vi "Magnetic Sweep 1.7.vi"() -> ()   [LabVIEW 2011]
uses:
  <vilib>/Math Plots/3D Math Plots/3D Scatter/3D Scatter XCtrl/3D Scatter.xctl
  <vilib>/Math Plots/3D Math Plots/3D Scatter/3D Scatter Datatype/Public/Plot Helper (Vector).vi
  <vilib>/Math Plots/3D Math Plots/3D Scatter/3D Scatter Datatype/3D Scatter Datatype.lvclass
panel:
  out "3D Scatter\n(ramp up)":refnum<class "3D Plot Datatype.lvclass">[](xcontrol)
  out "3D Scatter\n(ramp down)":refnum<class "3D Plot Datatype.lvclass">[](xcontrol)
  out "Heater":bool
  out "Persistent switch ready":bool
  out "error out 6":errorcluster
  in  "Temperature\nlower limite":dbl
  out "Ramping rate command":string
  out "Target field command":string
  out "error out 5":errorcluster
  in  "error out 4":errorcluster
  out "String":string="Persistent switch is not on"
  in  "Set parameter":bool
  out "status":string
  out "PID command":string
  out "setpoint command":string
  out "setpoint":dbl
  in  "stop":bool
  out "error out 3":errorcluster
  out "error out 2":errorcluster
  in  "Contour plot (ramp down)":path
  in  "Raw data (ramp down)":path
  out "Elapsed Time (s)":dbl
  out "Iteration":i32
  in  "error out":errorcluster
  out "Initial Temperature":string
  out "Zero field reached":bool
  out "Target field reached":bool
  in  "Temperature\nupper limite":dbl
  in  "Temperature\nramping step":dbl
  in  "Heater range":i16(ring) items=["High", "Medium", "Low"]
  in  "D gain":dbl
  in  "I gain":dbl
  in  "P gain":dbl
  in  "Contour plot (ramp up)":path
  out "Time elapsed":string
  in  "Timer":bool caption="Reset"
  in  "date format":enum16{"short", "long", "abbreviated"}(ring)
  in  "Save":bool
  in  "Raw data (ramp  up)":path
  out "Temperature vs Time":cluster{dbl[], dbl[]}(graph)
  out "current time":timestamp
  out "Magnetic\nField":cluster{dbl[], dbl[]}(graph)
  out "Current Resistance":string
  out "Current Temperature":string
  out "Current Field":string
  out "Status":string
  in  "Field Sweep":bool
  in  "Magnetic field\nRamp rate":dbl
  in  "Traget Field":dbl
  out "Init Response":string
  in  "error in (no error)":errorcluster
  in  "IP Address":string
  in  "Ramp":bool
  in  "Update":bool
  in  "Ramp to Zero":bool
  in  "P Switch":bool
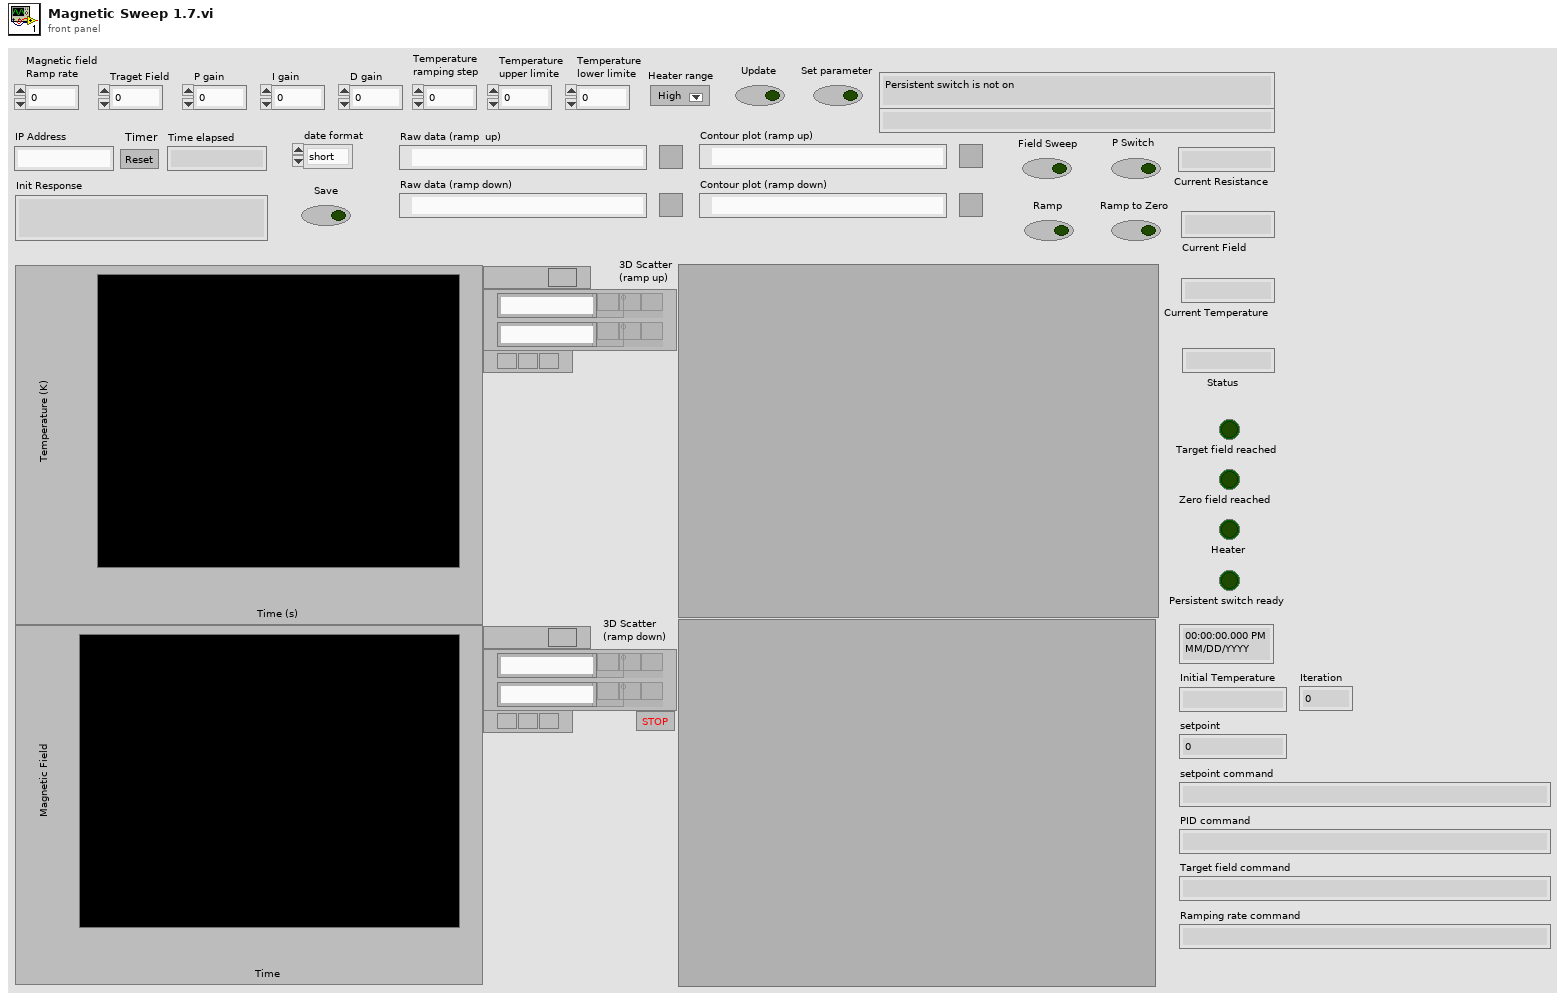
[diagram p1: front panel]
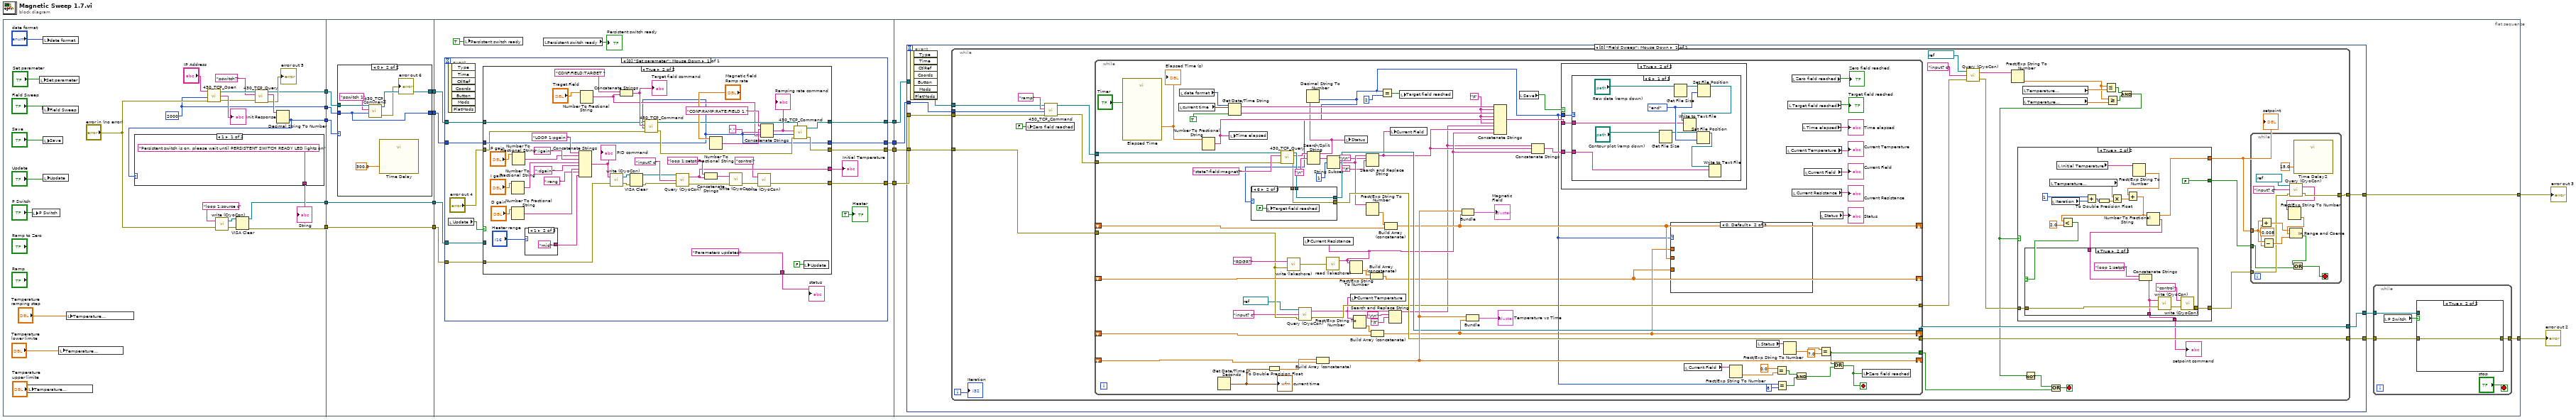
[diagram p0: block diagram]
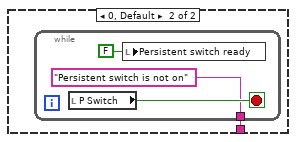
[diagram p2: hidden frame]
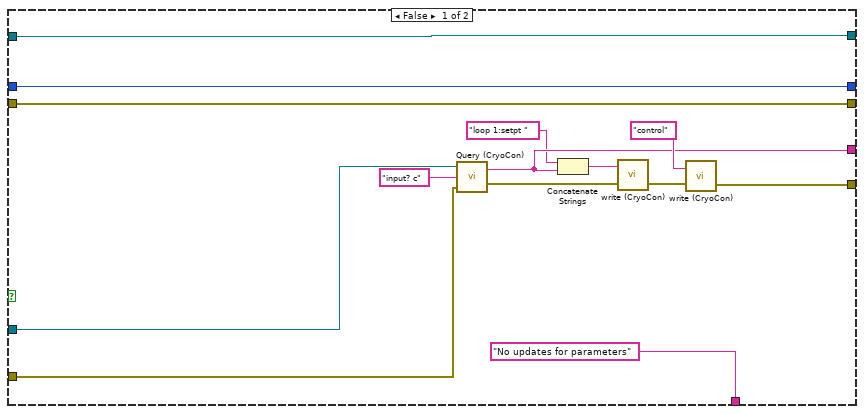
[diagram p4: hidden frame]
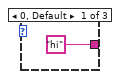
[diagram p5: hidden frame]
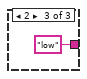
[diagram p6: hidden frame]
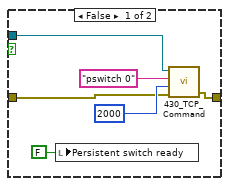
[diagram p7: hidden frame]
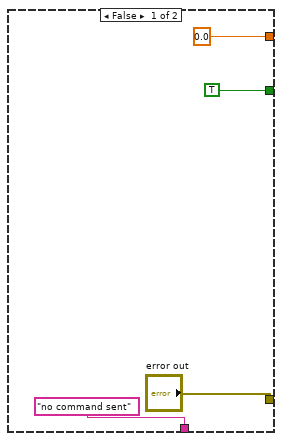
[diagram p8: hidden frame]
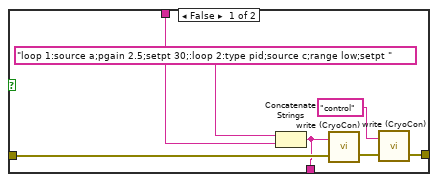
[diagram p9: hidden frame]
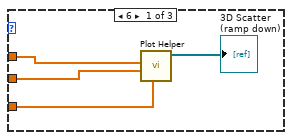
[diagram p10: hidden frame]
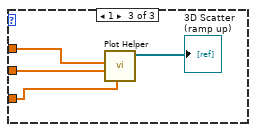
[diagram p11: hidden frame]
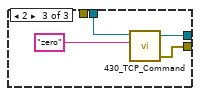
[diagram p13: hidden frame]
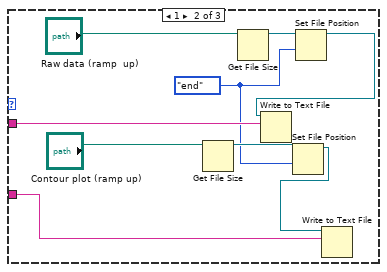
[diagram p15: hidden frame]
diagram:
  n1 = flat-sequence {
    tunnel: [w17] -> w9
    tunnel: [w20] -> w7
    tunnel: [w23] -> w5
    tunnel: [w21] -> w3
    tunnel: [w16] -> w1
    tunnel: w9 -> [w51]
    tunnel: [w49] -> w8
    tunnel: w7 -> [w50]
    tunnel: [w47] -> w6
    tunnel: w5 -> [w53]
    tunnel: [w53] -> w4
    tunnel: w3 -> [w52]
    tunnel: [w52] -> w2
    tunnel: w1 -> [w48]
    tunnel: w8 -> [w62]
    tunnel: w6 -> [w71]
    tunnel: w4 -> [w70]
    tunnel: [w69] -> w15
    tunnel: [w68] -> w12
    tunnel: [w67] -> w11
    tunnel: [w66] -> w10
    tunnel: w2 -> [w65]
    tunnel: w15 -> [w153]
    tunnel: [w152] -> w14
    tunnel: [w150] -> w13
    tunnel: w12 -> [w148]
    tunnel: w11 -> [w147]
    tunnel: w10 -> [w146]
    frame #0 {
      w20 = 2000 ("Timeout")
      n2 = local write "Temperature\nupper limite"("Temperature\nupper limite") -> ()
      n3 = local write "P Switch"("P Switch") -> ()
      n4 = local write "Set parameter"("Set parameter") -> ()
      n5 = local write "date format"("date format") -> ()
      n6 = local write "Field Sweep"("Field Sweep") -> ()
      n7 = local write "Save"("Save") -> ()
      n8 = local write "Update"("Update") -> ()
      n9 = local write "Temperature\nlower limite"("Temperature\nlower limite") -> ()
      n10 = local write "Temperature\nramping step"("Temperature\nramping step") -> ()
      n11 = call "430_TCP_Open.vi"("IP Address"="IP Address", "timeout ms (2000)"=w20, "error in (no error)"="error in (no error)") -> ("connection ID"=w30:refnum<k5>, "Init Response"=→"Init Response":string, "error out"=w29:errorcluster)  [unwired: 3 in]
      n12 = call "write (CryoCon).vi"("error in (no error)"="error in (no error)", "write buffer"="loop 1:source c") -> ("error out"=w25:errorcluster, "VISA resource name out"=w24:refnum<visa-resource-name>)
      n13 = VISA Clear(VISA resource name=w24, error in (no error)=w25) -> (VISA resource name out=w21:refnum<visa-resource-name>, error out=w23:errorcluster)
      n14 = call "430_TCP_Query.vi"("error in (no error)"=w29, "Command"="pswitch?", "connection ID"=w30) -> ("error out"=→"error out 5":errorcluster, "Response"=w27:string, "connection ID out"=w17:refnum<k5>)  [unwired: 4 in, 2 out]
      n15 = Decimal String To Number(string=w27) -> (number=w16:i32)  [unwired: 2 in, 1 out]
      n16 = case shown="1" w16 {
        tunnel: ["Persistent switch is on, please wait until PERSISTENT SWITCH READY LED lights on" w43] -> w22
        frame 1 {
        }
        frame 0, Default {
          n17 = while {
            tunnel: ["Persistent switch is not on"] -> w43
            stop <- w46 stop-if-true
            n18 = local read "P Switch"() -> (w46:bool)
            n19 = local write "Persistent switch ready"(FALSE ("Persistent switch ready")) -> ()
          }
        }
      }
      "String" <- w22
    }
    frame #1 {
      n20 = case shown="0" w48 {
        tunnel: w51 -> [w55 w61]
        tunnel: w50 -> [w54 w56]
        tunnel: [w55 w60] -> w49
        tunnel: [w54 w56] -> w47
        frame 1, Default {
        }
        frame 0 {
          n21 = call "430_TCP_Command.vi"("Timeout"=w56, "Command"="pswitch 1", "connection ID"=w61) -> ("error out"=→"error out 6":errorcluster, "connection ID out"=w60:refnum<k5>)  [unwired: 1 in, 1 out]
          n22 = call "Time Delay"("Delay Time (s)"=300.0) -> ()  [unwired: 10 in, 1 out]
        }
      }
    }
    frame #2 {
      n23 = event shown="[0] \"Set parameter\": Mouse Down" {
        selector: _ -> [_]
        dyn-events: _ -> [_]
        timeout: _ -> [_]
        tunnel: w62 -> [w84]
        tunnel: w71 -> [w83]
        tunnel: w70 -> [w82]
        tunnel: [w81] -> w69
        tunnel: [w80] -> w68
        tunnel: [w79] -> w67
        tunnel: [w78] -> w66
        tunnel: w65 -> [w74]
        event "Set parameter": Mouse Down {
          n24 = event-data() -> ()  [unwired: 1 in, 7 out]
          n25 = local read "Update"() -> (w75:bool)
          n26 = case shown="True" w75 {
            tunnel: w84 -> [w96 w140]
            tunnel: w83 -> [w97 w112]
            tunnel: w82 -> [w93 w119]
            tunnel: [w85 w100] -> w81
            tunnel: ["No updates for parameters" ("String") "Parameters updated" ("String")] -> w77
            tunnel: [w92 w114] -> w80
            tunnel: [w96 w113] -> w79
            tunnel: [w97 w112] -> w78
            tunnel: [w88 w104] -> w76
            tunnel: w74 -> [w94 _]
            tunnel: "error out 4" -> [w92 w99]
            frame False {
              n27 = call "Query (CryoCon).vi"("error in (no error)"=w93, "write buffer"="input? c", "VISA resource name 2"=w94) -> ("error out"=w86:errorcluster, "read buffer"=w88:string)
              n28 = Concatenate Strings("loop 1:setpt " ("write buffer"), w88) -> (w91:string)
              n29 = call "write (CryoCon).vi"("error in (no error)"=w86, "write buffer"=w91) -> ("error out"=w90:errorcluster)  [unwired: 1 out]
              n30 = call "write (CryoCon).vi"("error in (no error)"=w90, "write buffer"="control") -> ("error out"=w85:errorcluster)  [unwired: 1 out]
            }
            frame True {
              n31 = Number To Fractional String(number="I gain") -> (F-format string=w123:string)  [unwired: 3 in]
              n32 = Number To Fractional String(number="D gain") -> (F-format string=w121:string)  [unwired: 3 in]
              n33 = Number To Fractional String(number="P gain") -> (F-format string=w124:string)  [unwired: 3 in]
              n34 = case shown="1" "Heater range" {
                tunnel: ["hi" "mid" "low"] -> w116
                frame 0, Default {
                }
                frame 1 {
                }
                frame 2 {
                }
              }
              n35 = Concatenate Strings("LOOP 1:pgain " ("write buffer"), w124, ";igain " ("string"), w123, ";dgain " ("string"), w121, ";rang " ("string"), w116) -> (w120:string)
              "PID command" <- w120
              n36 = Number To Fractional String(number="Traget Field") -> (F-format string=w130:string)  [unwired: 3 in]
              n37 = call "write (CryoCon).vi"("error in (no error)"=w119, "write buffer"=w120) -> ("error out"=w111:errorcluster, "VISA resource name out"=w110:refnum<visa-resource-name>)
              n38 = Concatenate Strings("CONF:FIELD:TARGET ", w130) -> (w141:string)
              "Target field command" <- w141
              n39 = VISA Clear(VISA resource name=w110, error in (no error)=w111) -> (VISA resource name out=w107:refnum<visa-resource-name>, error out=w108:errorcluster)
              n40 = call "430_TCP_Command.vi"("error in (no error)"=w99, "Timeout"=w112, "Command"=w141, "connection ID"=w140) -> ("error out"=w139:errorcluster, "connection ID out"=w135:refnum<k5>)  [unwired: 1 out]
              n41 = call "Query (CryoCon).vi"("error in (no error)"=w108, "write buffer"="input? c", "VISA resource name 2"=w107) -> ("error out"=w106:errorcluster, "read buffer"=w104:string)
              n42 = Concatenate Strings("loop 1:setpt " ("write buffer"), w104) -> (w103:string)
              n43 = Number To Fractional String(number="Magnetic field\nRamp rate") -> (F-format string=w133:string)  [unwired: 3 in]
              n44 = call "write (CryoCon).vi"("error in (no error)"=w106, "write buffer"=w103) -> ("error out"=w102:errorcluster)  [unwired: 1 out]
              n45 = call "write (CryoCon).vi"("error in (no error)"=w102, "write buffer"="control") -> ("error out"=w100:errorcluster)  [unwired: 1 out]
              n46 = Concatenate Strings("CONF:RAMP:RATE:FIELD 1," ("string"), w133, "," ("string"), w130) -> (w136:string)
              "Ramping rate command" <- w136
              n47 = call "430_TCP_Command.vi"("error in (no error)"=w139, "Timeout"=w112, "Command"=w136, "connection ID"=w135) -> ("error out"=w114:errorcluster, "connection ID out"=w113:refnum<k5>)  [unwired: 1 out]
              n48 = local write "Update"(FALSE ("Update")) -> ()
            }
          }
          "Initial Temperature" <- w76
          "status" <- w77
          "Heater" <- TRUE ("Heater")
        }
      }
      n49 = local write "Persistent switch ready"(TRUE ("Persistent switch ready")) -> ()
      n50 = local read "Persistent switch ready"() -> (→"Persistent switch ready":bool)
    }
    frame #3 {
      n51 = event shown="[0] \"Field Sweep\": Mouse Down" {
        selector: _ -> [_]
        dyn-events: _ -> [_]
        timeout: _ -> [_]
        tunnel: w153 -> [w172]
        tunnel: [w171] -> w152
        tunnel: [w170] -> w151
        tunnel: [w169] -> w149
        tunnel: w148 -> [w168]
        tunnel: w147 -> [w167]
        tunnel: w146 -> [w166]
        event "Field Sweep": Mouse Down {
          n52 = event-data() -> ()  [unwired: 1 in, 7 out]
          n53 = while {
            tunnel: w172 -> [w201]
            tunnel: [w194] -> w171
            tunnel: [w193] -> w170
            tunnel: [w192] -> w169
            tunnel: w168 -> [w190]
            tunnel: w167 -> [w189]
            tunnel: w166 -> [w188]
            i -> [w198]
            stop <- w173 stop-if-true
            n54 = local write "Zero field reached"(FALSE ("Zero field reached")) -> ()
            n55 = call "430_TCP_Command.vi"("error in (no error)"=w190, "Timeout"=w188, "Command"="ramp", "connection ID"=w189) -> ("error out"=w202:errorcluster, "connection ID out"=w176:refnum<k5>)  [unwired: 1 out]
            n56 = while {
              shift-right: [w281] -> _
              shift-left: _ -> [w320]
              shift-right: [w268] -> _
              shift-left: _ -> [w325]
              shift-right: [w267] -> _
              shift-left: _ -> [w322]
              shift-right: [w317] -> _
              shift-left: _ -> [w264]
              tunnel: w202 -> [w307]
              tunnel: w176 -> [w306]
              tunnel: w201 -> [w278]
              tunnel: [w277] -> w186
              tunnel: [w289] -> w193
              tunnel: [w288] -> w192
              tunnel: [w251] -> w174
              stop <- w252 stop-if-true
              w311 = "\t"
              n57 = call "Elapsed Time"("Reset"="Timer") -> ("Elapsed Time (s)"=w301:dbl)  [unwired: 11 in, 7 out]
              "Elapsed Time (s)" <- w301
              n58 = local read "current time"() -> (w309:timestamp)
              n59 = local read "date format"() -> (w303:enum16{"short", "long", "abbreviated"})
              n60 = Number To Fractional String(number=w301) -> (F-format string=w304:string)  [unwired: 3 in]
              n61 = Get Date/Time In Seconds() -> (seconds since 1Jan1904=w300:timestamp)
              "current time" <- w300
              n62 = Get Date/Time String(date format (0)=w303, seconds (now)=w309, want seconds? (F)=TRUE) -> (date string=w313:string, time string=w312:string)
              n63 = local write "Time elapsed"(w304) -> ()
              n64 = To Double Precision Float(number=w300) -> (double precision float=w265:dbl)
              n65 = call "430_TCP_Query.vi"("error in (no error)"=w307, "Command"="state?;field:magnet?", "connection ID"=w306) -> ("error out"=w279:errorcluster, "Response"=w287:string, "connection ID out"=w290:refnum<k5>)  [unwired: 4 in, 2 out]
              n66 = call "write (lakeshore).vi"("error in (no error)"=w278, "write buffer"="RDGR?") -> ("error out"=w324:errorcluster)
              n67 = call "Query (CryoCon).vi"("error in (no error)"=w278, "write buffer"="input? c", "VISA resource name 2"=refnum<visa-resource-name> "COM3") -> ("error out"=w277:errorcluster, "read buffer"=w274:string)
              n68 = Search/Split String(string=w287, search string/char (-)="\n") -> (substring before match=w286:string, match + rest of string=w285:string)  [unwired: 1 in, 1 out]
              n69 = Decimal String To Number(string=w286) -> (number=w280:i32)  [unwired: 2 in, 1 out]
              n70 = case shown="6" w280 {
                tunnel: [w335 w337 w342] -> w288
                tunnel: w290 -> [w336 w339 w341]
                tunnel: [w336 w339 w340] -> w289
                tunnel: w279 -> [w335 w337 _]
                frame 0, Default {
                }
                frame 6 {
                  n71 = local write "Target field reached"(FALSE ("Target field reached")) -> ()
                }
                frame 2 {
                  n72 = call "430_TCP_Command.vi"("Command"="zero", "connection ID"=w341) -> ("error out"=w342:errorcluster, "connection ID out"=w340:refnum<k5>)  [unwired: 2 in, 1 out]
                }
              }
              n73 = Build Array (concatenate)(w265, w264) -> (w317:dbl[])
              n74 = call "read (lakeshore).vi"("error in (no error)"=w324) -> ("read buffer"=w266:string)  [unwired: 1 out]
              n75 = local write "Current Resistance"(w266) -> ()
              n76 = String Subset(string=w285, offset (0)=1) -> (substring=w271:string)  [unwired: 1 in]
              n77 = local write "Status"(w286) -> ()
              n78 = Fract/Exp String To Number(string=w266) -> (number=w318:dbl)  [unwired: 3 in, 1 out]
              n79 = local write "Current Temperature"(w274) -> ()
              n80 = Fract/Exp String To Number(string=w274) -> (number=w319:dbl)  [unwired: 3 in, 1 out]
              n81 = Search and Replace String(input string=w271, search string="\r\n", replace string="\t") -> (result string=w263:string)  [unwired: 5 in, 3 out]
              n82 = Fract/Exp String To Number(string=w271) -> (number=w321:dbl)  [unwired: 3 in, 1 out]
              n83 = Build Array (concatenate)(w318, w322) -> (w267:dbl[])
              n84 = Build Array (concatenate)(w319, w325) -> (w268:dbl[])
              n85 = Equal?(x=w280, y=2) -> (x = y?=w305:bool)
              n86 = Build Array (concatenate)(w321, w320) -> (w281:dbl[])
              n87 = Search and Replace String(input string=w274, search string="\r\n", replace string="\t") -> (result string=w262:string)  [unwired: 5 in, 3 out]
              n88 = local write "Current Field"(w263) -> ()
              n89 = local write "Target field reached"(w305) -> ()
              n90 = Bundle(w317, w281) -> (→"Magnetic\nField":cluster{dbl[], dbl[]})  [unwired: 1 in]
              n91 = Bundle(w317, w268) -> (→"Temperature vs Time":cluster{dbl[], dbl[]})  [unwired: 1 in]
              n92 = Concatenate Strings(w313, w311, w312, w311, w304, w311, w262, w263, w266) -> (w316:string)
              n93 = local read "Save"() -> (w299:bool)
              n94 = Concatenate Strings(w262, w263, w266) -> (w310:string)
              n95 = case shown="True" w299 {
                tunnel: w316 -> [_ w346]
                tunnel: w310 -> [_ w345]
                tunnel: w280 -> [_ w344]
                frame False {
                }
                frame True {
                  n96 = case shown="6" w344 {
                    tunnel: w346 -> [w348 w364 _]
                    tunnel: w345 -> [w347 w358 _]
                    frame 6 {
                      w354 = enum16{"start", "end", "current"}."end" ("from (0:start)")
                      n97 = Get File Size(file="Contour plot (ramp down)") -> (refnum out=w353:refnum<file>)  [unwired: 1 in, 2 out]
                      n98 = Get File Size(file="Raw data (ramp down)") -> (refnum out=w350:refnum<file>)  [unwired: 1 in, 2 out]
                      n99 = Set File Position(refnum=w353, from (0:start)=w354) -> (refnum out=w355:refnum<file>)  [unwired: 2 in, 1 out]
                      n100 = Set File Position(refnum=w350, from (0:start)=w354) -> (refnum out=w351:refnum<file>)  [unwired: 2 in, 1 out]
                      n101 = Write to Text File(file (use dialog)=w351, text=w348) -> ()  [unwired: 2 in, 3 out]
                      n102 = Write to Text File(file (use dialog)=w355, text=w347) -> ()  [unwired: 2 in, 3 out]
                    }
                    frame 1 {
                      w357 = enum16{"start", "end", "current"}."end" ("from (0:start)")
                      n103 = Get File Size(file="Contour plot (ramp up)") -> (refnum out=w359:refnum<file>)  [unwired: 1 in, 2 out]
                      n104 = Get File Size(file="Raw data (ramp  up)") -> (refnum out=w362:refnum<file>)  [unwired: 1 in, 2 out]
                      n105 = Set File Position(refnum=w359, from (0:start)=w357) -> (refnum out=w356:refnum<file>)  [unwired: 2 in, 1 out]
                      n106 = Set File Position(refnum=w362, from (0:start)=w357) -> (refnum out=w361:refnum<file>)  [unwired: 2 in, 1 out]
                      n107 = Write to Text File(file (use dialog)=w361, text=w364) -> ()  [unwired: 2 in, 3 out]
                      n108 = Write to Text File(file (use dialog)=w356, text=w358) -> ()  [unwired: 2 in, 3 out]
                    }
                    frame Default {
                    }
                  }
                }
              }
              n109 = case shown="0, Default" w280 {
                tunnel: w268 -> [w328 _ w331]
                tunnel: w281 -> [w327 _ w332]
                tunnel: w267 -> [w329 _ w333]
                frame 6 {
                  n110 = call-poly <vilib>:"Plot Helper.vi"("z vector"=w329, "y vector"=w327, "x vector"=w328) -> ("3D Plot lvclass Array out"=→"3D Scatter\n(ramp down)":refnum<class "3D Plot Datatype.lvclass">[])  [unwired: 3 in, 5 out]
                }
                frame 0, Default {
                }
                frame 1 {
                  n111 = call-poly <vilib>:"Plot Helper.vi"("z vector"=w333, "y vector"=w332, "x vector"=w331) -> ("3D Plot lvclass Array out"=→"3D Scatter\n(ramp up)":refnum<class "3D Plot Datatype.lvclass">[])  [unwired: 3 in, 5 out]
                }
              }
              n112 = local read "Current Field"() -> (w259:string)
              n113 = Fract/Exp String To Number(string=w259) -> (number=w257:dbl)  [unwired: 3 in, 1 out]
              n114 = local read "Status"() -> (w256:string)
              n115 = Equal?(x=0.0 ("y"), y=w257) -> (x = y?=w260:bool)
              n116 = Equal?(x=w280, y=8) -> (x = y?=w261:bool)
              n117 = Fract/Exp String To Number(string=w256) -> (number=w254:dbl)  [unwired: 3 in, 1 out]
              n118 = local read "Current Temperature"() -> (→"Current Temperature":string)
              n119 = local read "Target field reached"() -> (→"Target field reached":bool)
              n120 = local read "Zero field reached"() -> (→"Zero field reached":bool)
              n121 = local read "Current Resistance"() -> (→"Current Resistance":string)
              n122 = And(x=w260, y=w261) -> (x .and. y?=w253:bool)
              n123 = local read "Time elapsed"() -> (→"Time elapsed":string)
              n124 = local read "Current Field"() -> (→"Current Field":string)
              n125 = Equal?(x=w254, y=7.0) -> (x = y?=w251:bool)
              n126 = local read "Status"() -> (→"Status":string)
              n127 = Or(x=w251, y=w253) -> (x .or. y?=w252:bool)
              n128 = local write "Zero field reached"(w252) -> ()
            }
            n129 = call "Query (CryoCon).vi"("error in (no error)"=w186, "write buffer"="input? c", "VISA resource name 2"=refnum<visa-resource-name> "COM3") -> ("error out"=w185:errorcluster, "read buffer"=w184:string)
            n130 = Fract/Exp String To Number(string=w184) -> (number=w182:dbl)  [unwired: 3 in, 1 out]
            n131 = local read "Temperature\nupper limite"() -> (w195:dbl)
            n132 = local read "Temperature\nlower limite"() -> (w181:dbl)
            n133 = Less Or Equal?(x=w182, y=w195) -> (x <= y?=w179:bool)
            n134 = Greater Or Equal?(x=w182, y=w181) -> (x >= y?=w180:bool)
            n135 = And(x=w179, y=w180) -> (x .and. y?=w178:bool)
            n136 = case shown="True" w178 {
              tunnel: w185 -> [_ w235]
              tunnel: ["error out" w225] -> w200
              tunnel: [0.0 w223] -> w199
              tunnel: ["no command sent" w229] -> w191
              tunnel: [TRUE FALSE] -> w177
              frame False {
              }
              frame True {
                n137 = local read "Temperature\nramping step"() -> (w231:dbl)
                n138 = local read "Iteration"() -> (w228:i32)
                n139 = local read "Initial Temperature"() -> (w234:string)
                n140 = Add(x=1, y=w228) -> (x+y=w227:i32)
                n141 = To Double Precision Float(number=w227) -> (double precision float=w230:dbl)
                n142 = Multiply(x=w231, y=w230) -> (x*y=w232:dbl)
                n143 = Fract/Exp String To Number(string=w234) -> (number=w233:dbl)  [unwired: 3 in, 1 out]
                n144 = Add(x=w233, y=w232) -> (x+y=w223:dbl)
                n145 = Less?(x=w223, y=2.0) -> (x < y?=w221:bool)
                n146 = Number To Fractional String(number=w223) -> (F-format string=w236:string)  [unwired: 3 in]
                n147 = case shown="True" w221 {
                  tunnel: w236 -> [w242 w249]
                  tunnel: w235 -> [w241 w248]
                  tunnel: [w238 w247] -> w229
                  tunnel: [w240 w246] -> w225
                  frame False {
                    n148 = Concatenate Strings("loop 1:source a;pgain 2.5;setpt 30;:loop 2:type pid;source c;range low;setpt " ("write buffer"), w242) -> (w238:string)
                    n149 = call "write (CryoCon).vi"("error in (no error)"=w241, "write buffer"=w238) -> ("error out"=w237:errorcluster)  [unwired: 1 out]
                    n150 = call "write (CryoCon).vi"("error in (no error)"=w237, "write buffer"="control") -> ("error out"=w240:errorcluster)  [unwired: 1 out]
                  }
                  frame True {
                    n151 = Concatenate Strings("loop 1:setpt " ("write buffer"), w249) -> (w247:string)
                    n152 = call "write (CryoCon).vi"("error in (no error)"=w248, "write buffer"=w247) -> ("error out"=w245:errorcluster)  [unwired: 1 out]
                    n153 = call "write (CryoCon).vi"("error in (no error)"=w245, "write buffer"="control") -> ("error out"=w246:errorcluster)  [unwired: 1 out]
                  }
                }
              }
            }
            "setpoint" <- w199
            "setpoint command" <- w191
            n154 = Not(x=w178) -> (.not. x?=w175:bool)
            n155 = Or(x=w175, y=w174) -> (x .or. y?=w173:bool)
            n156 = while {
              tunnel: w200 -> [w209]
              tunnel: w199 -> [w215]
              tunnel: [w208] -> w194
              tunnel: w177 -> [w205]
              stop <- w203 stop-if-true
              w212 = 0.008 ("y")
              n157 = Add(x=w215, y=w212) -> (x+y=w214:dbl)
              n158 = Subtract(x=w215, y=w212) -> (x-y=w213:dbl)
              n159 = call "Query (CryoCon).vi"("error in (no error)"=w209, "write buffer"="input? c", "VISA resource name 2"=refnum<visa-resource-name> "COM3") -> ("error out"=w208:errorcluster, "read buffer"=w207:string)
              n160 = Fract/Exp String To Number(string=w207) -> (number=w216:dbl)  [unwired: 3 in, 1 out]
              n161 = In Range and Coerce(upper limit=w214, x=w216, lower limit=w213) -> (In Range?=w204:bool)  [unwired: 1 out]
              n162 = Or(x=w204, y=w205) -> (x .or. y?=w203:bool)
              n163 = call "Time Delay2"("Delay Time (s)"=15.0) -> ()  [unwired: 10 in, 1 out]
            }
            "Iteration" <- w198
          }
        }
      }
      n164 = while {
        tunnel: w151 -> [w158]
        tunnel: [w156] -> w150
        tunnel: w149 -> [w155]
        stop <- "stop" stop-if-true
        n165 = local read "P Switch"() -> (w157:bool)
        n166 = case shown="True" w157 {
          tunnel: w158 -> [w163 _]
          tunnel: [w161 w165] -> w156
          tunnel: w155 -> [w160 w165]
          frame False {
            n167 = local write "Persistent switch ready"(FALSE ("Persistent switch ready")) -> ()
            n168 = call "430_TCP_Command.vi"("error in (no error)"=w160, "Timeout"=2000, "Command"="pswitch 0", "connection ID"=w163) -> ("error out"=w161:errorcluster)  [unwired: 2 out]
          }
          frame True {
          }
        }
      }
    }
  }
  "error out 2" <- w13
  "error out 3" <- w14
